vi "move.vi"(8 "error in (no error)":errorcluster, 11 "DL090409StageScaffold in":refnum<class "StageMH110930Scientifica.lvclass">) -> (0 "error out":errorcluster, 3 "DL090409StageScaffold out":refnum<class "StageMH110930Scientifica.lvclass">)   [LabVIEW 2010, in "StageMH110930Scientifica.lvclass"]
uses:
  StageMH110930Scientifica.lvclass
  StageDL090409Scaffold/StageDL090409Scaffold/StageDL090409Scaffold.lvclass
  common/classes/ErrorController/ErrorController/class_data.vi
  common/classes/ErrorController/ErrorController/ErrorController.lvclass
  common/classes/SpaceVector/SpaceVector/SpaceVector.lvclass
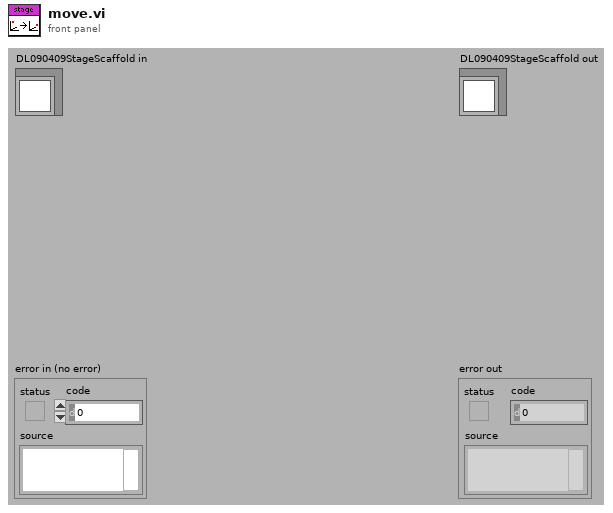
[diagram p1: front panel]
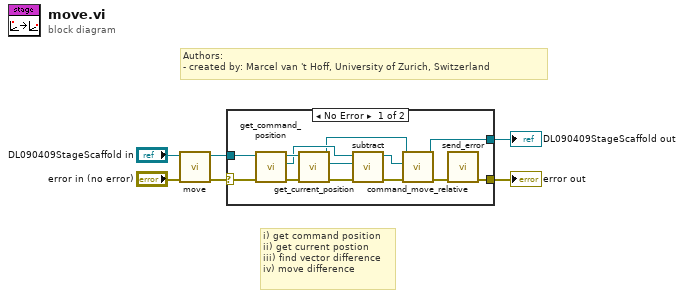
[diagram p0: block diagram]
diagram:
  # "i) get command position\nii) get current postion\niii) find vector difference\niv) move difference"
  # "Authors: \n- created by: Marcel van 't Hoff, University of Zurich, Switzerland"
  n1 = call-parent "move.vi"("error in (no error)"="error in (no error)", "DL090409StageScaffold in"="DL090409StageScaffold in") -> ("error out"=w4:errorcluster, "DL090409StageScaffold out"=w3:refnum<class "StageMH110930Scientifica.lvclass">)  [unwired: 8 in]
  n2 = case shown="No Error" w4 {
    selector: w4 -> [w15 w21]
    tunnel: [w18 w21] -> w2
    tunnel: [w8 w20] -> w1
    tunnel: w3 -> [w19 w20]
    frame No Error {
      n3 = call-dynamic "get_command_position.vi"("error in (no error)"=w15, "DL090409StageScaffold.lvclass in"=w19) -> ("error out"=w17:errorcluster, "SpaceVector.lvclass"=w14:refnum<class "SpaceVector.lvclass">, "DL090409StageScaffold.lvclass out"=w16:refnum<class "StageMH110930Scientifica.lvclass">)  [unwired: 7 out]
      n4 = call-dynamic "get_current_position.vi"("error in (no error)"=w17, "DL090409StageScaffold.lvclass in"=w16) -> ("error out"=w12:errorcluster, "current position"=w13:refnum<class "SpaceVector.lvclass">, "DL090409StageScaffold.lvclass out"=w9:refnum<class "StageMH110930Scientifica.lvclass">)  [unwired: 7 in]
      n5 = call "subtract.vi"("error in (no error)"=w12, "subtrahend"=w13, "SpaceVector in"=w14) -> ("error out"=w10:errorcluster, "SpaceVector out"=w11:refnum<class "SpaceVector.lvclass">)  [unwired: 7 in]
      n6 = call-dynamic "command_move_relative.vi"("error in (no error)"=w10, "target  position"=w11, "StageMH110930Scientifica in"=w9) -> ("error out"=w7:errorcluster, "StageMH110930Scientifica out"=w8:refnum<class "StageMH110930Scientifica.lvclass">)  [unwired: 7 in]
      n7 = call "send_error.vi"("error in (no error)"=w7) -> ("error out"=w18:errorcluster)  [unwired: 10 in]
    }
    frame Error {
    }
  }
  "error out" <- w2
  "DL090409StageScaffold out" <- w1
